vi "Decrement Clients Count.vi"(8 "error in (no error)":errorcluster, 11 "Data Value Reference in":refnum<data-value>) -> (0 "error out":errorcluster, 2 "Clients count":i32, 3 "Data Value Reference out":refnum<data-value>)   [LabVIEW 2015, in "Modbus Module runtime.lvclass"]
uses:
  Modbus Module runtime.lvclass
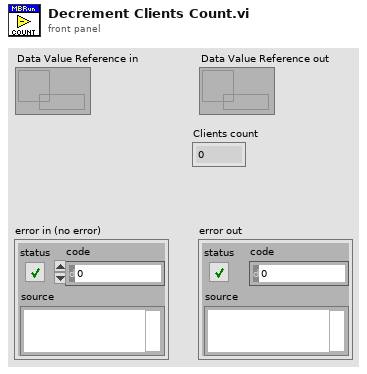
[diagram p1: front panel]
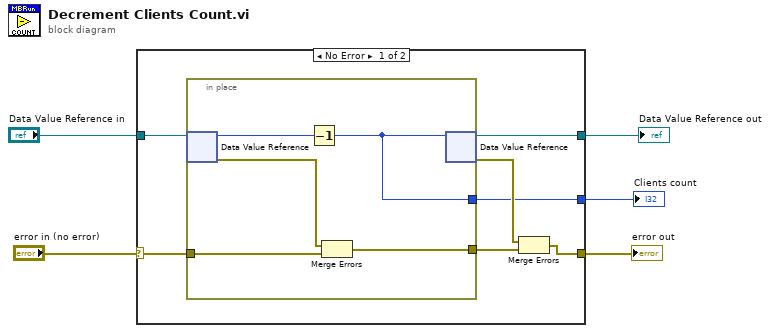
[diagram p0: block diagram]
diagram:
  n1 = case shown="No Error" "error in (no error)" {
    selector: "error in (no error)" -> [w10 w19]
    tunnel: [w7 w19] -> w4
    tunnel: "Data Value Reference in" -> [w12 w18]
    tunnel: [w11 w18] -> w2
    tunnel: [w6 _] -> w1
    frame No Error {
      n2 = in-place {
        in-place-border: w10 -> [w15]
        in-place-border: [w14] -> w8
        in-place-border: [w13] -> w6
        n3 = in-place-dvr #1(w12) -> (w17:i32, w16:errorcluster)
        n4 = Decrement(x=w17) -> (x-1=w13:i32)
        n5 = Merge Errors(w16, w15) -> (w14:errorcluster)
        n6 = in-place-dvr #1(w13) -> (w11:refnum<data-value>, w9:errorcluster)
      }
      n7 = Merge Errors(w9, w8) -> (w7:errorcluster)
    }
    frame Error {
    }
  }
  "error out" <- w4
  "Data Value Reference out" <- w2
  "Clients count" <- w1
